vi "Autofrettage Main.vi"() -> ()   [LabVIEW 2025]
doc: "This VI can be used as a launcher VI for the main application or as a debugging tool.\n_____\nBased on DQMH Dev Tools: Project Template 7.1.0.1503."
uses:
  Libraries/Autofrettage UI/Autofrettage UI.lvlib
  Libraries/Launcher Support/Launcher Support.lvlib
panel:
  in  "Launch Settings Editor API Tester":bool
  in  "Launch Logger API Tester":bool
  in  "Launch Acquisition API Tester":bool
  in  "Launch CML UI API Tester":bool
  out "Command Line Arguments":string[](array[string])
  out "Module Running?":bool
  out "Status":string
  out "error out":errorcluster
  in  "Stop Module":bool
  in  "Start Module":bool
  # "See the Build_Final_EXE bookmarks on the diagram for instructions on using this VI as a launcher for an EXE."
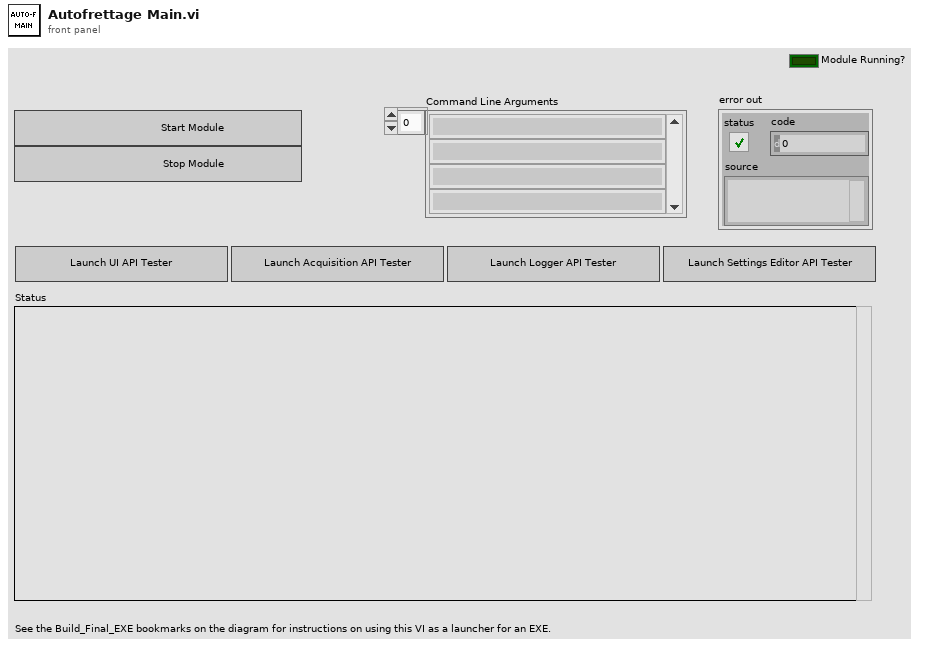
[diagram p1: front panel]
types:
  T1 = enum32{"invalid app kind", "Development System", "Run Time System", "Student Edition", "Embedded LabVIEW", "Evaluation", "Custom"}
  T2 = typedef "Autofrettage UI.lvlib/Broadcast Events--cluster.ctl" = cluster{"Module Did Init":refnum<user-event>, "Status Updated":refnum<user-event>, "Error Reported":refnum<user-event>, "Module Did Stop":refnum<user-event>, "Update Module Execution Status":refnum<user-event>}
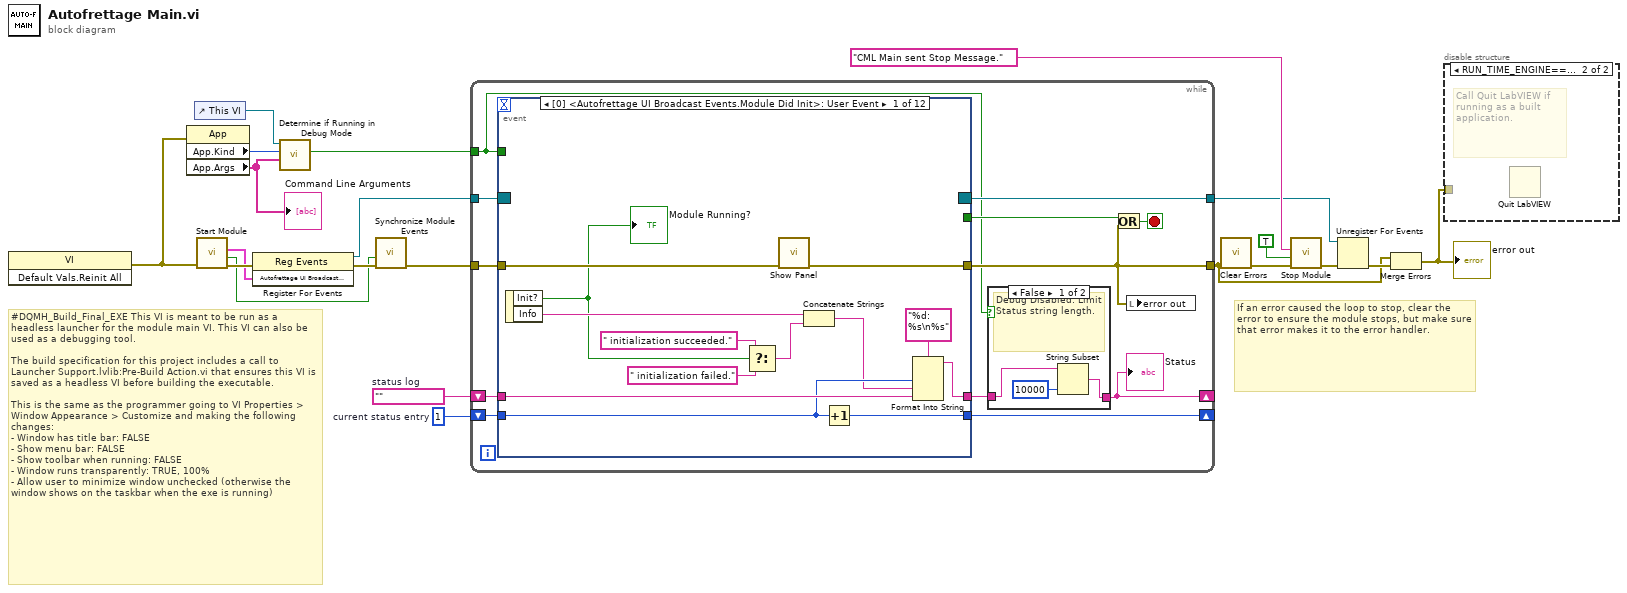
[diagram p0: block diagram]
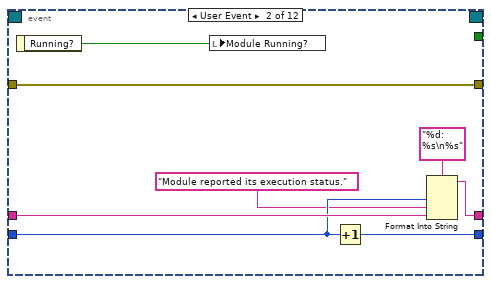
[diagram p3: hidden frame]
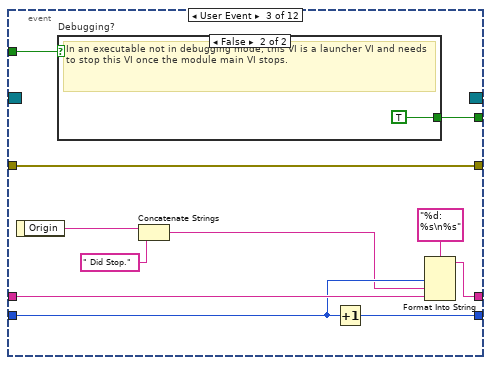
[diagram p4: hidden frame]
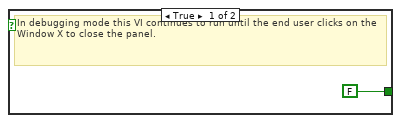
[diagram p5: hidden frame]
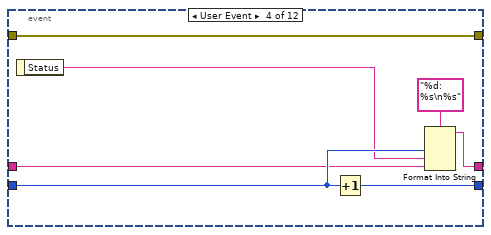
[diagram p6: hidden frame]
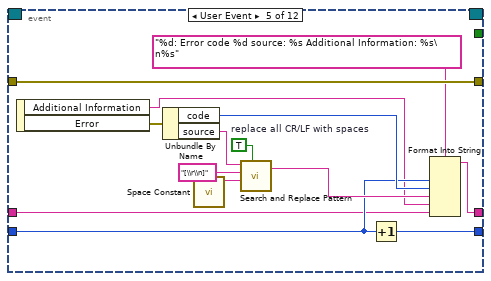
[diagram p7: hidden frame]
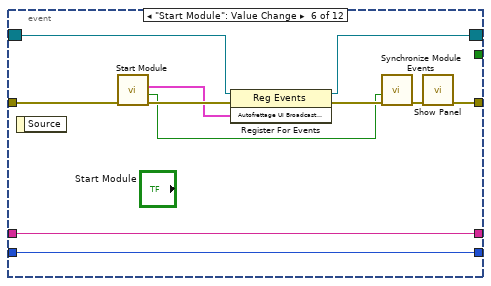
[diagram p8: hidden frame]
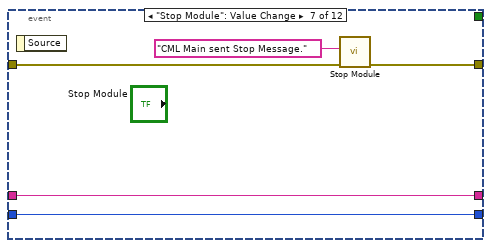
[diagram p9: hidden frame]
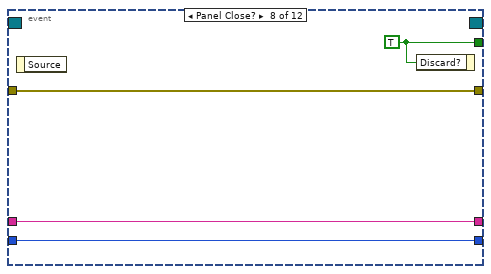
[diagram p10: hidden frame]
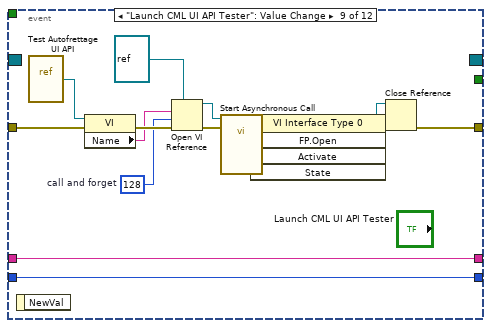
[diagram p11: hidden frame]
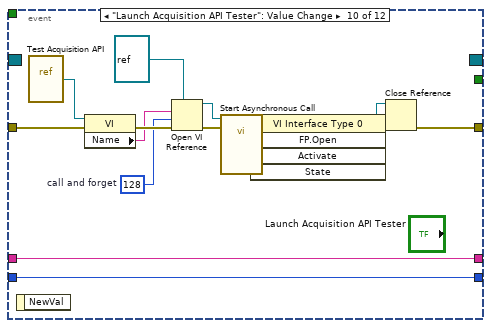
[diagram p12: hidden frame]
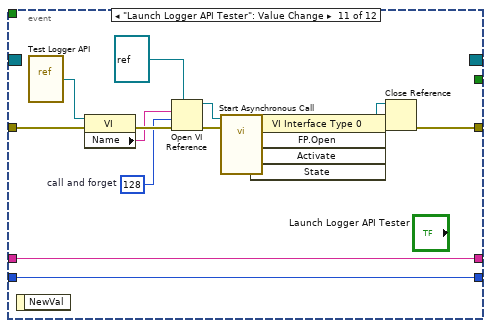
[diagram p13: hidden frame]
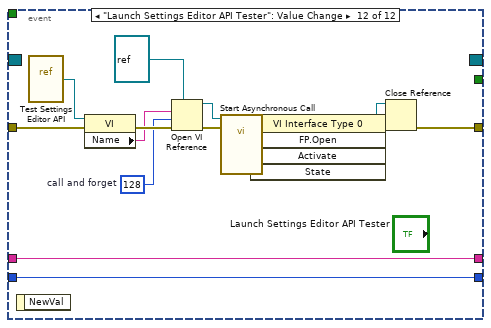
[diagram p14: hidden frame]
diagram:
  w10 = 1  # current status entry
  w11 = ""  # status log
  # "#DQMH_Build_Final_EXE This VI is meant to be run as a headless launcher for the module main VI. This VI can also be used as a debugging tool. \n\nThe build specification for this project includes a call to Launcher Support.lvlib:Pre-Build Action.vi that ensures this VI is saved as a headless VI before building the executable.\n\nThis is the same as the programmer going to VI Properties > Window Appearance > Customize and making the following changes:\n- Window has title bar: FALSE\n- Show menu bar: FALSE\n- Show toolbar when running: FALSE\n- Window runs transparently: TRUE, 100%\n- Allow user to minimize window unchecked (otherwise the window shows on the taskbar when the exe is running)"
  # "If an error caused the loop to stop, clear the error to ensure the module stops, but make sure that error makes it to the error handler."
  n1 = invoke on="Invoke Node" class="VI" method="Default Vals.Reinit All"() -> (error out=w13:errorcluster)  [unwired: 3 in, 2 out]
  n2 = property on="Property Node" class="App"(error in=w13) -> ("App.Kind"=w1:T1, "App.Args"=w4:string[])  [unwired: 1 in, 2 out]
  "Command Line Arguments" <- w4
  n3 = control-ref of="This VI"() -> (w3:refnum<vi>)
  n4 = call "Start Module.vi"("error in"=w13) -> ("error out"=w17:errorcluster, "Wait for Event Sync?"=w7:bool, "Autofrettage UI Broadcast Events"=w6:T2)  [unwired: 6 in, 2 out]
  n5 = register-events(error in=w17, w6) -> (reference out=w5:refnum<event-registration>, error out=w18:errorcluster)  [unwired: 1 in]
  n6 = call "Determine if Running in Debug Mode.vi"("App.Args"=w4, "App.Kind"=w1, "Launcher VI ref"=w3) -> ("Debug mode?"=w2:bool)  [unwired: 8 in]
  n7 = call "Synchronize Module Events.vi"("error in"=w18, "Wait for Event Sync?"=w7) -> ("error out"=w15:errorcluster)  [unwired: 9 in]
  n8 = while {
    tunnel: w5 -> [w31]
    tunnel: [w32] -> w14
    shift-right: [w23] -> _
    shift-left: w11 -> [w28]
    shift-right: [w27] -> _
    shift-left: w10 -> [w29]
    tunnel: w15 -> [w33]
    tunnel: [w25] -> w9
    tunnel: w2 -> [w22]
    stop <- w26 stop-if-true
    n9 = event shown="[0] <Autofrettage UI Broadcast Events.Module Did Init>: User Event" {
      selector: w31 -> [_ _ _ _ _ w94 _ _ _ _ _ _]
      dyn-events: [_ _ _ _ _ w93 _ _ _ _ _ _] -> w25
      timeout: _ -> [_ _ _ _ _ _ _ _ _ _ _ _]
      tunnel: [_ _ w60 _ _ _ _ w111 _ _ _ _] -> w30
      tunnel: [w49 w58 w69 w78 w92 w99 w108 w112 w115 w130 w145 w160] -> w32
      tunnel: w29 -> [w46 w55 w66 w74 w82 w97 w105 w109 w125 w140 w155 w170]
      tunnel: w28 -> [w47 w56 w67 w73 w80 w98 w106 w110 w126 w141 w156 w171]
      tunnel: [w44 w53 w64 w75 w83 w98 w106 w110 w126 w141 w156 w171] -> w24
      tunnel: [w45 w54 w65 w77 w81 w97 w105 w109 w125 w140 w155 w170] -> w27
      tunnel: w33 -> [w50 w58 w69 w78 w92 w101 w107 w112 w127 w142 w157 w172]
      tunnel: w22 -> [_ _ w59 _ _ _ _ _ _ _ _ _]
      event User Event {
        n10 = event-data() -> ("Init?"=w41:bool, "Info"=w43:string)  [unwired: 1 in]
        "Module Running?" <- w41
        n11 = Select(t=" initialization succeeded.", s=w41, f=" initialization failed.") -> (s? t:f=w38:string)
        n12 = call "Show Panel.vi"("error in"=w50) -> ("error out"=w49:errorcluster)  [unwired: 10 in]
        n13 = Concatenate Strings(w43, w38) -> (w42:string)
        n14 = Increment(x=w46) -> (x+1=w45:i32)
        n15 = Format Into String(format string="%d: %s\n%s", w46, w42, w47) -> (resulting string=w44:string)  [unwired: 2 in, 1 out]
      }
      event User Event {
        n16 = event-data() -> ("Running?"=w51:bool)  [unwired: 1 in]
        n17 = local write "Module Running?"(w51) -> ()
        n18 = Increment(x=w55) -> (x+1=w54:i32)
        n19 = Format Into String(format string="%d: %s\n%s", w55, "Module reported its execution status.", w56) -> (resulting string=w53:string)  [unwired: 2 in, 1 out]
      }
      event User Event {
        n20 = event-data() -> ("Origin"=w63:string)  [unwired: 1 in]
        n21 = case "Debugging?" shown="False" w59 {
          tunnel: [FALSE ("Discard?") TRUE ("Discard?")] -> w60
          frame True {
            # "In debugging mode this VI continues to run until the end user clicks on the Window X to close the panel."
          }
          frame False {
            # "In an executable not in debugging mode, this VI is a launcher VI and needs to stop this VI once the module main VI stops."
          }
        }
        n22 = Concatenate Strings(w63, " Did Stop.") -> (w62:string)
        n23 = Increment(x=w66) -> (x+1=w65:i32)
        n24 = Format Into String(format string="%d: %s\n%s", w66, w62, w67) -> (resulting string=w64:string)  [unwired: 2 in, 1 out]
      }
      event User Event {
        n25 = event-data() -> ("Status"=w72:string)  [unwired: 1 in]
        n26 = Increment(x=w74) -> (x+1=w77:i32)
        n27 = Format Into String(format string="%d: %s\n%s", w74, w72, w73) -> (resulting string=w75:string)  [unwired: 2 in, 1 out]
      }
      event User Event {
        w87 = TRUE  # replace all CR/LF with spaces
        n28 = event-data() -> ("Additional Information"=w79:string, "Error"=w91:errorcluster)  [unwired: 1 in]
        n29 = Unbundle By Name(w91) -> ("code"=w84:i32, "source"=w85:string)
        n30 = call <vilib>:"Space Constant.vi"() -> ("String"=w88:string)
        n31 = call <vilib>:"Search and Replace Pattern.vi"("string"=w85, "regular expression (\"\")"="[\\r\\n]" ("regular expression (\"\")"), "replace string (\"\")"=w88, "replace all? (F)"=w87) -> ("result string"=w86:string)  [unwired: 1 in, 1 out]
        n32 = Increment(x=w82) -> (x+1=w81:i32)
        n33 = Format Into String(format string="%d: Error code %d source: %s Additional Information: %s\n%s", w82, w84, w86, w79, w80) -> (resulting string=w83:string)  [unwired: 2 in, 1 out]
      }
      event "Start Module": Value Change {
        n34 = event-data() -> ()  [unwired: 1 in, 1 out]
        n35 = call "Start Module.vi"("error in"=w101) -> ("error out"=w102:errorcluster, "Wait for Event Sync?"=w96:bool, "Autofrettage UI Broadcast Events"=w95:T2)  [unwired: 6 in, 2 out]
        n36 = register-events(reference=w94, error in=w102, w95) -> (reference out=w93:refnum<event-registration>, error out=w103:errorcluster)
        n37 = call "Synchronize Module Events.vi"("error in"=w103, "Wait for Event Sync?"=w96) -> ("error out"=w100:errorcluster)  [unwired: 9 in]
        n38 = call "Show Panel.vi"("error in"=w100) -> ("error out"=w99:errorcluster)  [unwired: 10 in]
      }
      event "Stop Module": Value Change {
        n39 = event-data() -> ()  [unwired: 1 in, 1 out]
        n40 = call "Stop Module.vi"("error in"=w107, "Origin"="CML Main sent Stop Message.") -> ("error out"=w108:errorcluster)  [unwired: 9 in]
      }
      event Panel Close? {
        w111 = TRUE ("Discard?")
        n41 = event-data() -> ()  [unwired: 1 in, 1 out]
        n42 = event-data ("Event Filter Node")("Discard?"=w111) -> ()  [unwired: 1 in, 1 out]
      }
      event "Launch CML UI API Tester": Value Change {
        w113 = 128  # call and forget
        n43 = event-data() -> ()  [unwired: 1 in, 1 out]
        n44 = vi-ref "Test Autofrettage UI API.vi"() -> (w123:refnum<vi>)
        n45 = property class="VI"(reference=w123, error in=w127) -> (error out=w124:errorcluster, "Name"=w121:string)  [unwired: 1 out]
        n46 = Open VI Reference(type specifier VI Refnum (for type only)=refnum<vi> refnum, vi path=w121, options=w113, error in (no error)=w124) -> (vi reference=w118:refnum<vi>, error out=w122:errorcluster)  [unwired: 2 in]
        n47 = call-by-ref "Start Asynchronous Call"(reference=w118, error in=w122) -> (reference out=w116:refnum<vi>, error out=w119:errorcluster)  [unwired: 12 in]
        n48 = invoke class="VI Interface Type 0" method="FP.Open"(reference=w116, error in=w119) -> (reference out=w114:refnum<vi>, error out=w117:errorcluster)  [unwired: 3 in, 3 out]
        n49 = Close Reference(reference=w114, error in (no error)=w117) -> (error out=w115:errorcluster)
      }
      event "Launch Acquisition API Tester": Value Change {
        w128 = 128  # call and forget
        n50 = event-data() -> ()  [unwired: 1 in, 1 out]
        n51 = vi-ref "Test Acquisition API.vi"() -> (w138:refnum<vi>)
        n52 = property class="VI"(reference=w138, error in=w142) -> (error out=w139:errorcluster, "Name"=w136:string)  [unwired: 1 out]
        n53 = Open VI Reference(type specifier VI Refnum (for type only)=refnum<vi> refnum, vi path=w136, options=w128, error in (no error)=w139) -> (vi reference=w133:refnum<vi>, error out=w137:errorcluster)  [unwired: 2 in]
        n54 = call-by-ref "Start Asynchronous Call"(reference=w133, error in=w137) -> (reference out=w131:refnum<vi>, error out=w134:errorcluster)  [unwired: 12 in]
        n55 = invoke class="VI Interface Type 0" method="FP.Open"(reference=w131, error in=w134) -> (reference out=w129:refnum<vi>, error out=w132:errorcluster)  [unwired: 3 in, 3 out]
        n56 = Close Reference(reference=w129, error in (no error)=w132) -> (error out=w130:errorcluster)
      }
      event "Launch Logger API Tester": Value Change {
        w143 = 128  # call and forget
        n57 = event-data() -> ()  [unwired: 1 in, 1 out]
        n58 = vi-ref "Test Logger API.vi"() -> (w153:refnum<vi>)
        n59 = property class="VI"(reference=w153, error in=w157) -> (error out=w154:errorcluster, "Name"=w151:string)  [unwired: 1 out]
        n60 = Open VI Reference(type specifier VI Refnum (for type only)=refnum<vi> refnum, vi path=w151, options=w143, error in (no error)=w154) -> (vi reference=w148:refnum<vi>, error out=w152:errorcluster)  [unwired: 2 in]
        n61 = call-by-ref "Start Asynchronous Call"(reference=w148, error in=w152) -> (reference out=w146:refnum<vi>, error out=w149:errorcluster)  [unwired: 12 in]
        n62 = invoke class="VI Interface Type 0" method="FP.Open"(reference=w146, error in=w149) -> (reference out=w144:refnum<vi>, error out=w147:errorcluster)  [unwired: 3 in, 3 out]
        n63 = Close Reference(reference=w144, error in (no error)=w147) -> (error out=w145:errorcluster)
      }
      event "Launch Settings Editor API Tester": Value Change {
        w158 = 128  # call and forget
        n64 = event-data() -> ()  [unwired: 1 in, 1 out]
        n65 = vi-ref "Test Settings Editor API.vi"() -> (w168:refnum<vi>)
        n66 = property class="VI"(reference=w168, error in=w172) -> (error out=w169:errorcluster, "Name"=w166:string)  [unwired: 1 out]
        n67 = Open VI Reference(type specifier VI Refnum (for type only)=refnum<vi> refnum, vi path=w166, options=w158, error in (no error)=w169) -> (vi reference=w163:refnum<vi>, error out=w167:errorcluster)  [unwired: 2 in]
        n68 = call-by-ref "Start Asynchronous Call"(reference=w163, error in=w167) -> (reference out=w161:refnum<vi>, error out=w164:errorcluster)  [unwired: 12 in]
        n69 = invoke class="VI Interface Type 0" method="FP.Open"(reference=w161, error in=w164) -> (reference out=w159:refnum<vi>, error out=w162:errorcluster)  [unwired: 3 in, 3 out]
        n70 = Close Reference(reference=w159, error in (no error)=w162) -> (error out=w160:errorcluster)
      }
    }
    n71 = case shown="False" w22 {
      tunnel: w24 -> [w36 w37]
      tunnel: [w35 w37] -> w23
      frame False {
        # "Debug Disabled. Limit Status string length."
        n72 = String Subset(string=w36, length (rest)=10000 ("length (rest)")) -> (substring=w35:string)  [unwired: 1 in]
      }
      frame True {
        # "Debug Enabled. Do not limit Status string length."
      }
    }
    "Status" <- w23
    n73 = Or(x=w30, y=w32) -> (x .or. y?=w26:bool)
    n74 = local write "error out"(w32) -> ()
  }
  n75 = call <vilib>:"Clear Errors.vi"("error in (no error)"=w14) -> ("error out"=w19:errorcluster)  [unwired: 5 in, 1 out]
  n76 = call "Stop Module.vi"("error in"=w19, "Wait for Module to Stop? (F)"=TRUE ("Wait for Module to stop?"), "Origin"="CML Main sent Stop Message.") -> ("error out"=w20:errorcluster)  [unwired: 8 in]
  n77 = Unregister For Events(event registration refnum=w9, error in=w20) -> (error out=w21:errorcluster)
  n78 = Merge Errors(w14, w21) -> (w16:errorcluster)
  "error out" <- w16
  n79 = disable-structure "Conditional Disable Structure" shown="RUN_TIME_ENGINE==True" {
    disable-tunnel: w16 -> [_ _]
    frame condition #0 (active) {
    }
    frame condition #1 {
      # "Call Quit LabVIEW if running as a built application."
      n80 = Quit LabVIEW() -> ()  [unwired: 1 in]
    }
  }
